vi "Create.vi"(7 "visa open timeout":u32, 8 "error in":errorcluster, 10 "access mode":T1 items=["VISA Defaults"=0, "Exclusive Lock"=1, "Load Configured Settings"=4], 11 "instrument type id":string) -> (0 "error out":errorcluster, 3 "session factory out":refnum<class "Session Factory.lvclass">)   [LabVIEW 2020, in "NI Session Management VISA.lvlib" / "Session Factory.lvclass"]
uses:
  Session Factory.lvclass
  <vilib>/Instr/_visa.llb/VISA Open Access Mode.ctl
  Session Factory.lvclass/Session Factory.ctl
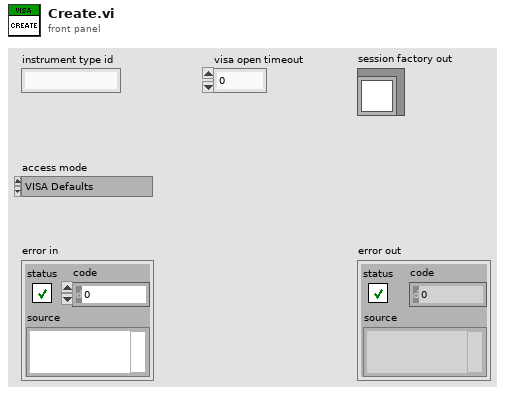
[diagram p1: front panel]
types:
  T1 = typedef "VISA Open Access Mode.ctl" = u32
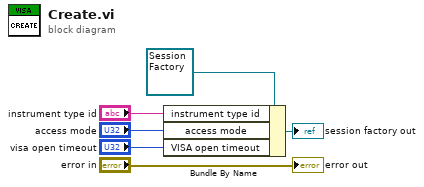
[diagram p0: block diagram]
diagram:
  n1 = Bundle By Name(cluster=refnum<class "Session Factory.lvclass"> refnum ("Instrument in"), "instrument type id"="instrument type id", "access mode"="access mode", "VISA open timeout"="visa open timeout") -> (→"session factory out":refnum<class "Session Factory.lvclass">)
  "error out" <- "error in"
